vi "Configure.vi"(8 "error in (no error)":errorcluster, 11 "Retiga in":refnum<class "Retiga.lvclass">) -> (0 "error out":errorcluster, 2 "cancelled?":bool, 3 "Retiga out":refnum<class "Retiga.lvclass">)   [LabVIEW 2012, in "Retiga.lvclass"]
doc: "The configure method configures the details for the RabbitMQ connection, the observers and the mapping script.\n\nIn the derived class, make a call to the parent for setting these parameters."
uses:
  Retiga.lvclass
  dependencies/ImageReg/Registration method.ctl
  dependencies/ImageReg/BinarizationParameters.ctl
  dependencies/ImageReg/Gaussian blur parameters.ctl
  dependencies/ImageReg/Edge and object parameters.ctl
  <vilib>/Utility/miscctls.llb/LVPointTypeDef.ctl
  Retiga.lvclass/Retiga.ctl
  <vilib>/Distrio/Murmex/Murmex/Murmex.lvclass
panel:
  in  "button:call_parent":bool
  in  "button:cancel":bool
  in  "button:ok":bool
  in  "Tab Control":T1(tab)
  in  "saturation limit":dbl
  in  "stage component":string
  in  "micron equivalent of pixel":dbl[unit]
  in  "max x pixel displacement":dbl
  in  "max pixel discrepancy":dbl
  in  "max y pixel displacement":dbl
  in  "max physical displacement":dbl[unit]
  in  "brightness threshold":sgl
  in  "min physical displacement":dbl[unit]
  in  "temperature":dbl
  in  "invert image?":bool
  in  "pixel size":sgl[unit]
  in  "Registration method":T2
  in  "Binarization parameters":T3={"threshold percentage"=95.0, "equalize?"=FALSE, "Method (clustering)"=0} {"Method (clustering)" items=["clustering", "entropy", "metric", "moments", "inter-class variance"]}
  in  "Gaussian blur parameters":T4={"large sigma"=20.0, "small sigma"=4.0, "equalize?"=FALSE}
  in  "Edge and object Parameters":T5={"Canny Edge Parameters"={"Sigma"=1.0, "HThresh"=0.7, "LThres"=0.2, "WindowSize"=9}, "Smoothing parameters"={"X Size"=3, "Y Size"=3, "% Tolerance"=40}, "Dilation iteration"=1, "Object recognition parameters"={"Objects"=0, "Threshold"=128, "Reject Border"=FALSE, "Fill Holes"=FALSE, "Min Object Size"=FALSE, "Min Size"=3, "Max Object Size"=FALSE, "Max Size"=100, "Show Search Area"=FALSE, "Show Center"=TRUE, "Show Bounding Box"=TRUE}} {"Object recognition parameters"."Objects" items=["Bright Objects", "Dark Objects"]; "Object recognition parameters"."Threshold" min=1 max=999999999 step=1; "Object recognition parameters"."Max Size" min=1 max=999999999 step=1; "Object recognition parameters"."Min Size" min=1 max=999999999 step=1; "Canny Edge Parameters"."LThres" min=0 max=1 format="%.2f"; "Canny Edge Parameters"."HThresh" min=0 max=1 format="%.2f"; "Canny Edge Parameters"."Sigma" min=0 max=1 format="%.2f"}
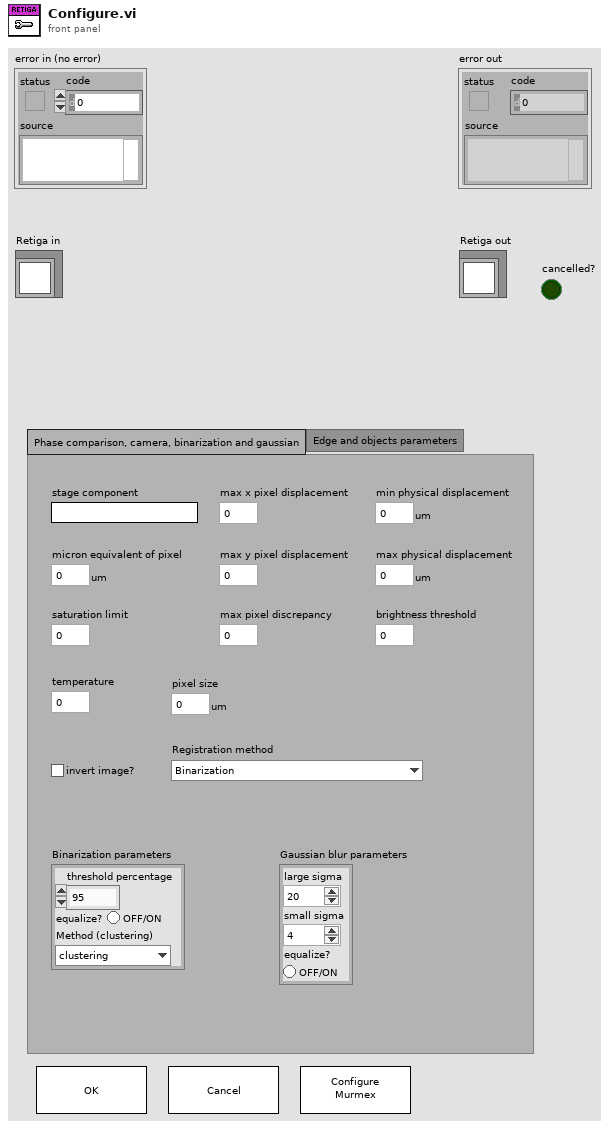
[diagram p1: front panel]
types:
  T1 = enum32{"Phase comparison, camera, binarization and gaussian", "Edge and objects parameters"}
  T2 = typedef "Registration method.ctl" = enum16{"Binarization", "Difference of Gaussians", "Edges Detection", "Gaussians and Binarization", "Edges and Gaussians", "Edges and Binarization", "All"}
  T3 = typedef "BinarizationParameters.ctl" = cluster{"threshold percentage":dbl, "equalize?":bool, "Method (clustering)":i32}
  T4 = typedef "Gaussian blur parameters.ctl" = cluster{"large sigma":sgl, "small sigma":sgl, "equalize?":bool}
  T5 = typedef "Edge and object parameters.ctl" = cluster{"Canny Edge Parameters":cluster{"Sigma":sgl, "HThresh":sgl, "LThres":sgl, "WindowSize":i32}, "Smoothing parameters":cluster{"X Size":i32, "Y Size":i32, "% Tolerance":i32}, "Dilation iteration":i32, "Object recognition parameters":cluster{"Objects":u16, "Threshold":i32, "Reject Border":bool, "Fill Holes":bool, "Min Object Size":bool, "Min Size":i32, "Max Object Size":bool, "Max Size":i32, "Show Search Area":bool, "Show Center":bool, "Show Bounding Box":bool}}
  T6 = typedef "LVPointTypeDef.ctl" = cluster{"Horizontal":i16, "Vertical":i16}
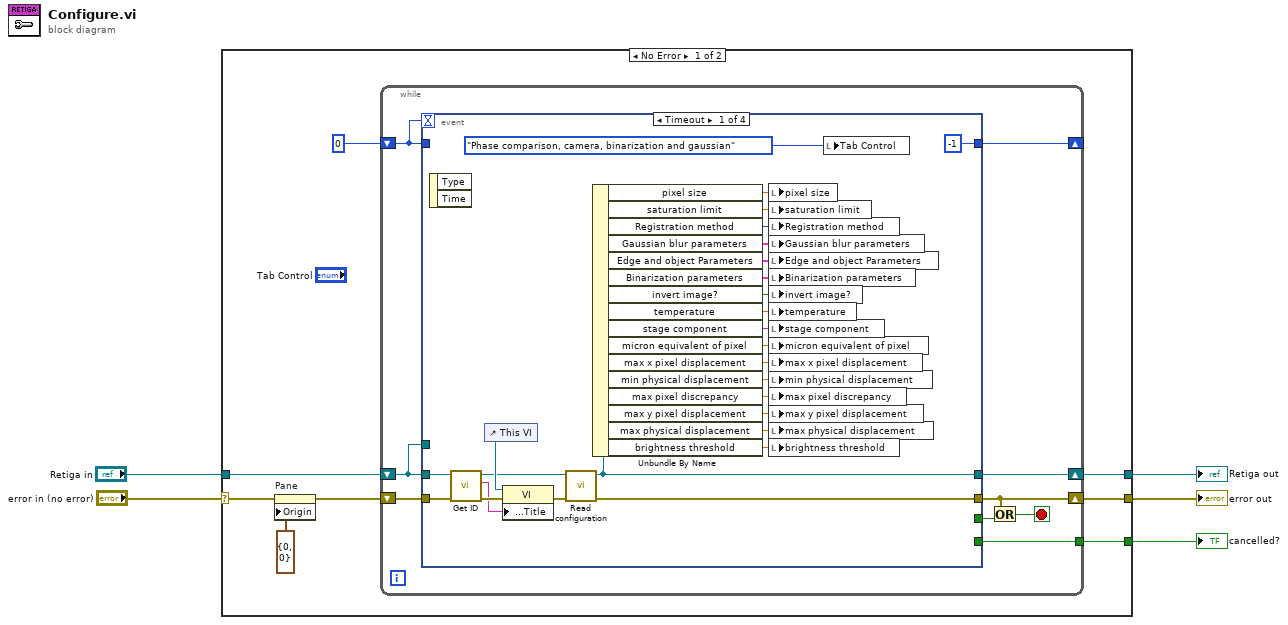
[diagram p0: block diagram]
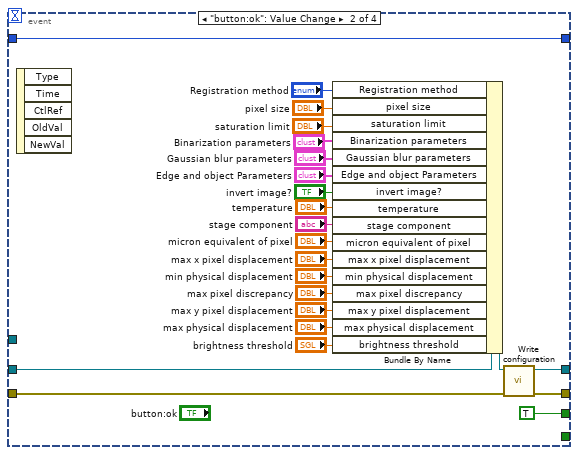
[diagram p2: hidden frame]
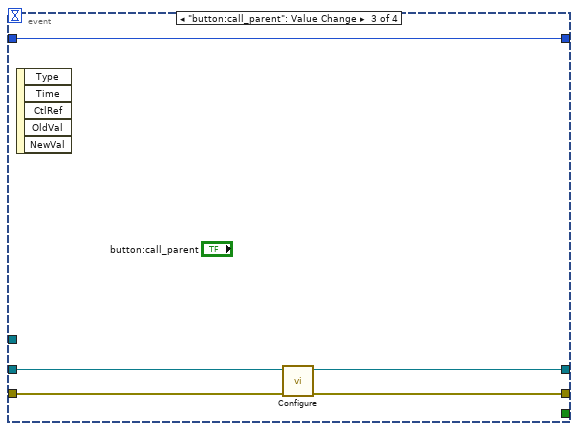
[diagram p3: hidden frame]
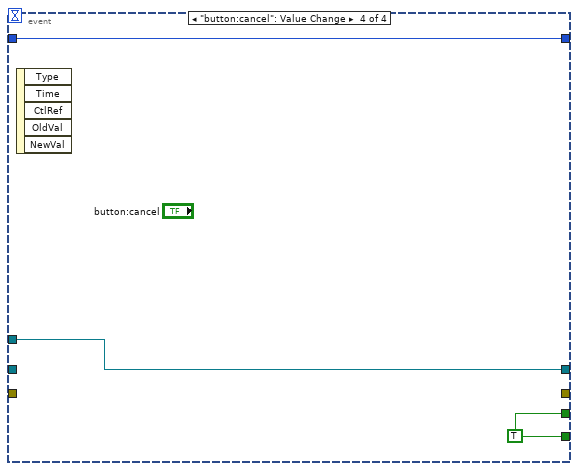
[diagram p4: hidden frame]
diagram:
  n1 = case shown="No Error" "error in (no error)" {
    selector: "error in (no error)" -> [w12 w81]
    tunnel: [w7 w82] -> w4
    tunnel: "Retiga in" -> [w10 w82]
    tunnel: [w8 w81] -> w2
    tunnel: [w6 _] -> w1
    frame No Error {
      n2 = property on="Pane" class="Pane"(error in=w12, "Origin"=T6 {"Horizontal"=0, "Vertical"=0}) -> (error out=w11:errorcluster)  [unwired: 1 in, 1 out]
      n3 = while {
        shift-right: [w16] -> w8
        shift-left: w11 -> [w22]
        shift-right: [w18] -> w7
        shift-left: w10 -> [w21]
        shift-right: [w19] -> _
        shift-left: 0 -> [w20]
        tunnel: [w14] -> w6
        stop <- w15 stop-if-true
        n4 = event shown="[0] Timeout" {
          selector: _ -> [_ _ _ _]
          dyn-events: _ -> [_ _ _ _]
          timeout: w20 -> [_ _ _ _]
          tunnel: w22 -> [w43 w72 w77 _]
          tunnel: w21 -> [w42 w70 w76 _]
          tunnel: w21 -> [_ _ _ w80]
          tunnel: w20 -> [_ w57 w73 w78]
          tunnel: [-1 w57 w73 w78] -> w19
          tunnel: [w40 w71 w74 _] -> w16
          tunnel: [w41 w68 w75 w80] -> w18
          tunnel: [_ TRUE ("y") _ w79] -> w17
          tunnel: [_ _ _ w79] -> w14
          event Timeout {
            n5 = event-data() -> ()  [unwired: 1 in, 2 out]
            n6 = call <vilib>:"Get ID.vi"("error in (no error)"=w43, "Murmex in"=w42) -> ("error out"=w48:errorcluster, "component id"=w44:string, "Murmex out"=w45:refnum<class "Retiga.lvclass">)  [unwired: 7 in]
            n7 = control-ref of="This VI"() -> (w47:refnum<vi>)
            n8 = property class="VI"(reference=w47, error in=w48, "Front Panel.Title"=w44) -> (error out=w46:errorcluster)  [unwired: 1 out]
            n9 = call <vilib>:"Read configuration.vi"("error in (no error)"=w46, "Murmex in"=w45) -> ("error out"=w40:errorcluster, "Murmex out"=w41:refnum<class "Retiga.lvclass">)  [unwired: 7 in, 1 out]
            n10 = Unbundle By Name(w41) -> ("pixel size"=w28:sgl[unit], "saturation limit"=w27:dbl, "Registration method"=w26:T2, "Gaussian blur parameters"=w24:T4, "Edge and object Parameters"=w23:T5, "Binarization parameters"=w25:T3, "invert image?"=w30:bool, "temperature"=w34:dbl, "stage component"=w33:string, "micron equivalent of pixel"=w35:dbl[unit], "max x pixel displacement"=w32:dbl, "min physical displacement"=w37:dbl[unit], "max pixel discrepancy"=w38:dbl, "max y pixel displacement"=w39:dbl, "max physical displacement"=w31:dbl[unit], "brightness threshold"=w36:sgl)
            n11 = local write "pixel size"(w28) -> ()
            n12 = local write "saturation limit"(w27) -> ()
            n13 = local write "Registration method"(w26) -> ()
            n14 = local write "Gaussian blur parameters"(w24) -> ()
            n15 = local write "Edge and object Parameters"(w23) -> ()
            n16 = local write "Binarization parameters"(w25) -> ()
            n17 = local write "invert image?"(w30) -> ()
            n18 = local write "temperature"(w34) -> ()
            n19 = local write "stage component"(w33) -> ()
            n20 = local write "micron equivalent of pixel"(w35) -> ()
            n21 = local write "max x pixel displacement"(w32) -> ()
            n22 = local write "min physical displacement"(w37) -> ()
            n23 = local write "max pixel discrepancy"(w38) -> ()
            n24 = local write "max y pixel displacement"(w39) -> ()
            n25 = local write "max physical displacement"(w31) -> ()
            n26 = local write "brightness threshold"(w36) -> ()
            n27 = local write "Tab Control"(T1."Phase comparison, camera, binarization and gaussian" ("Tab Control")) -> ()
          }
          event "button:ok": Value Change {
            n28 = event-data() -> ()  [unwired: 1 in, 5 out]
            n29 = Bundle By Name(cluster=w70, "Registration method"="Registration method", "pixel size"="pixel size", "saturation limit"="saturation limit", "Binarization parameters"="Binarization parameters", "Gaussian blur parameters"="Gaussian blur parameters", "Edge and object Parameters"="Edge and object Parameters", "invert image?"="invert image?", "temperature"="temperature", "stage component"="stage component", "micron equivalent of pixel"="micron equivalent of pixel", "max x pixel displacement"="max x pixel displacement", "min physical displacement"="min physical displacement", "max pixel discrepancy"="max pixel discrepancy", "max y pixel displacement"="max y pixel displacement", "max physical displacement"="max physical displacement", "brightness threshold"="brightness threshold") -> (w69:refnum<class "Retiga.lvclass">)
            n30 = call <vilib>:"Write configuration.vi"("error in (no error)"=w72, "Murmex in"=w69) -> ("error out"=w71:errorcluster, "Murmex out"=w68:refnum<class "Retiga.lvclass">)  [unwired: 8 in]
          }
          event "button:call_parent": Value Change {
            n31 = event-data() -> ()  [unwired: 1 in, 5 out]
            n32 = call-parent "Configure.vi"("error in (no error)"=w77, "Murmex in"=w76) -> ("error out"=w74:errorcluster, "Murmex out"=w75:refnum<class "Retiga.lvclass">)  [unwired: 7 in, 1 out]
          }
          event "button:cancel": Value Change {
            w79 = TRUE
            n33 = event-data() -> ()  [unwired: 1 in, 5 out]
          }
        }
        n34 = Or(x=w16, y=w17) -> (x .or. y?=w15:bool)
      }
    }
    frame Error {
    }
  }
  "error out" <- w2
  "Retiga out" <- w4
  "cancelled?" <- w1
